vi "Get Library Path.vi"() -> (0 "Path":path)   [LabVIEW 2017, in "libssh2.lvlib"]
uses:
  libssh2.lvlib
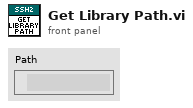
[diagram p1: front panel]
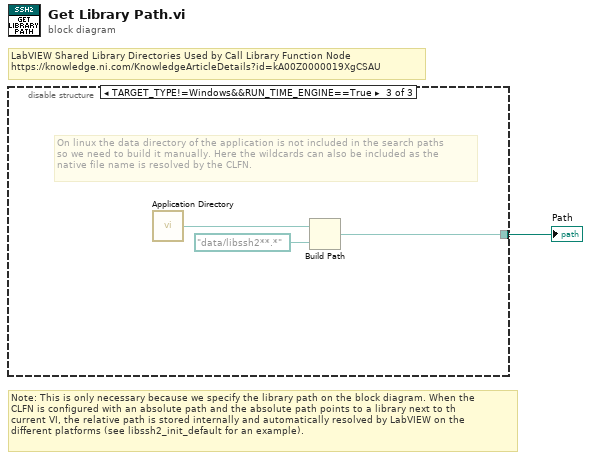
[diagram p0: block diagram]
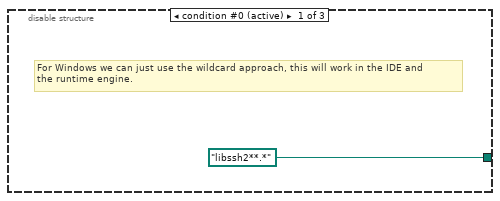
[diagram p2: hidden frame]
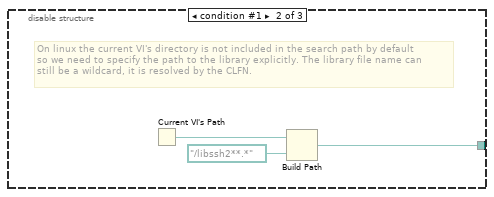
[diagram p3: hidden frame]
diagram:
  # "Note: This is only necessary because we specify the library path on the block diagram. When the\nCLFN is configured with an absolute path and the absolute path points to a library next to th\ncurrent VI, the relative path is stored internally and automatically resolved by LabVIEW on the\ndifferent platforms (see libssh2_init_default for an example)."
  # "LabVIEW Shared Library Directories Used by Call Library Function Node\nhttps://knowledge.ni.com/KnowledgeArticleDetails?id=kA00Z0000019XgCSAU"
  n1 = disable-structure shown="TARGET_TYPE!=Windows&&RUN_TIME_ENGINE==True" {
    disable-tunnel: [path "libssh2**.*" w3 w6] -> w1
    frame condition #0 (active) {
      # "For Windows we can just use the wildcard approach, this will work in the IDE and\nthe runtime engine."
    }
    frame condition #1 {
      # "On linux the current VI's directory is not included in the search path by default\nso we need to specify the path to the library explicitly. The library file name can\nstill be a wildcard, it is resolved by the CLFN."
      n2 = Current VI's Path() -> (path=w4:path)
      n3 = Build Path(base path=w4, name or relative path=path "../libssh2**.*") -> (appended path=w3:path)
    }
    frame condition #2 {
      # "On linux the data directory of the application is not included in the search paths\nso we need to build it manually. Here the wildcards can also be included as the\nnative file name is resolved by the CLFN."
      n4 = call <vilib>:"Application Directory.vi"() -> ("Application Directory"=w7:path)
      n5 = Build Path(base path=w7, name or relative path=path "data/libssh2**.*") -> (appended path=w6:path)
    }
  }
  "Path" <- w1
